vi "Get 'M' RefNum.vi"(8 "error in (no error)":errorcluster, 11 "This VI":refnum<vi>) -> (0 "error out":errorcluster, 3 "'M' Refnum":refnum<vi>)   [LabVIEW 2014]
doc: "This VI takes a reference to a VI and returns the 'M' text decoration reference. It also will make the 'M' invisible by default.\n\nAuthor: Erik Johnson, National Instruments"
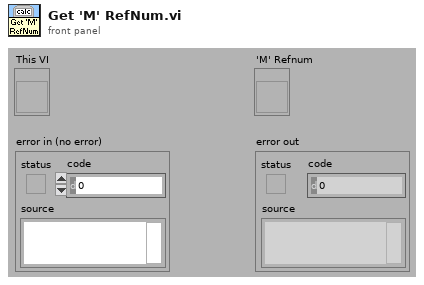
[diagram p1: front panel]
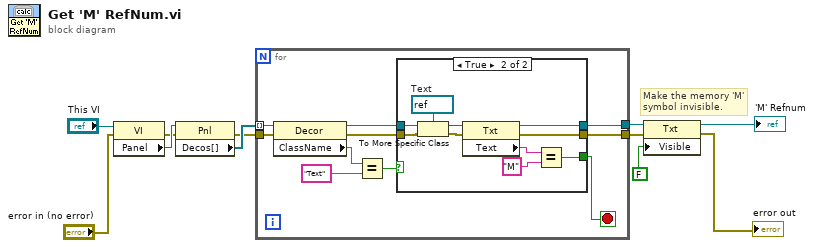
[diagram p0: block diagram]
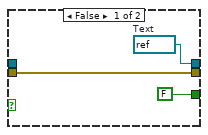
[diagram p2: hidden frame]
diagram:
  # "Make the memory 'M' symbol invisible."
  n1 = property class="VI"(reference="This VI", error in="error in (no error)") -> (error out=w7:errorcluster, "Panel"=w10:refnum<vi>)  [unwired: 1 out]
  n2 = property class="Pnl"(reference=w10, error in=w7) -> (error out=w6:errorcluster, "Decos[]"=w11:refnum<vi>[])  [unwired: 1 out]
  n3 = for {
    tunnel: w11 -> [w21] mode=indexing
    tunnel: w6 -> [w18]
    tunnel: [w14] -> w4
    tunnel: [w12] -> w3
    stop <- w13 stop-if-true
    n4 = property class="Decor"(reference=w21, error in=w18) -> (reference out=w16:refnum<vi>, error out=w15:errorcluster, "ClassName"=w19:string)
    n5 = Equal?(x=w19, y="Text") -> (x = y?=w17:bool)
    n6 = case shown="True" w17 {
      tunnel: w16 -> [_ w33]
      tunnel: w15 -> [w23 w32]
      tunnel: [w23 w27] -> w14
      tunnel: [FALSE w26] -> w13
      tunnel: [w22 w25] -> w12
      frame False {
        w22 = refnum<vi> refnum  # Text
      }
      frame True {
        w34 = refnum<vi> refnum  # Text
        n7 = To More Specific Class(target class=w34, reference=w33, error in=w32) -> (specific class reference=w30:refnum<vi>, error out=w31:errorcluster)
        n8 = property class="Txt"(reference=w30, error in=w31) -> (reference out=w25:refnum<vi>, error out=w27:errorcluster, "Text"=w29:string)
        n9 = Equal?(x=w29, y="M") -> (x = y?=w26:bool)
      }
    }
  }
  n10 = property class="Txt"(reference=w3, error in=w4, "Visible"=FALSE) -> (reference out=→"'M' Refnum":refnum<vi>, error out=→"error out":errorcluster)
